vi "Add New Floor.vi"(1 "Rock Grid in":set{cdb}(c389)) -> (0 "Rock Grid out":set{cdb}(c389))   [LabVIEW 2020, in "AoC 2022.lvlib"]
uses:
  AoC 2022.lvlib
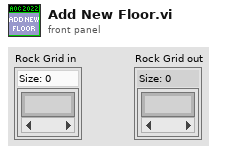
[diagram p1: front panel]
types:
  T1 = cluster{"Left":i16, "Top":i16, "Right":i16, "Bottom":i16}
  T2 = cluster{"Left":i32, "Top":i32, "Right":i32, "Bottom":i32}
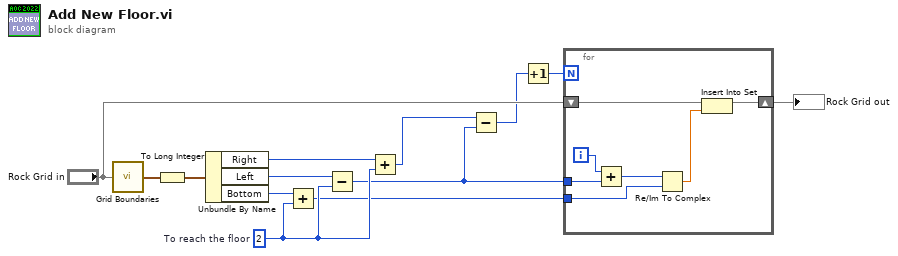
[diagram p0: block diagram]
diagram:
  w13 = 2  # To reach the floor
  n1 = call "Grid Boundaries.vi"("Grid"="Rock Grid in") -> ("Bounds"=w4:T1)
  n2 = To Long Integer(number=w4) -> (32bit integer=w7:T2)
  n3 = Unbundle By Name(w7) -> ("Right"=w5:i32, "Left"=w3:i32, "Bottom"=w1:i32)
  n4 = Add(x=w1, y=w13) -> (x+y=w8:i32)
  n5 = Subtract(x=w3, y=w13) -> (x-y=w10:i32)
  n6 = Add(x=w5, y=w13) -> (x+y=w9:i32)
  n7 = Subtract(x=w9, y=w10) -> (x-y=w6:i32)
  n8 = Increment(x=w6) -> (x+1=w2:i32)
  n9 = for {
    N: w2 -> [_]
    tunnel: w8 -> [w20]
    tunnel: w10 -> [w15]
    shift-right: [w17] -> w12
    shift-left: "Rock Grid in" -> [w19]
    i -> [w14]
    n10 = Add(x=w14, y=w15) -> (x+y=w16:i32)
    n11 = Re/Im To Complex(1:w20, 2:w16) -> (0:w18:cdb)
    n12 = Insert Into Set(10:w18, 11:w19) -> (3:w17:set{cdb})  [unwired: 1 out]
  }
  "Rock Grid out" <- w12
